vi "PH_VacuumControl.set modified data.vi"(0 "i ref in":refnum<vi>, 2 "i attribute":T1={"GUI Refs"={"Exit"=refnum, "Set Unit"=refnum, "Device found"=refnum, "Busy"=refnum, "State"=refnum, "Delete"=refnum, "Channels"=refnum, "Channel Name"=refnum, "Trend"=refnum, "Logarithmic"=refnum, "Limit reached"=refnum, "Channel Name 1 MT"=refnum, "Channel Name 2 MT"=refnum, "Trend MT"=refnum, "Logarithmic MT"=refnum, "Limit reached MT"=refnum}, "Device found"=FALSE, "Busy"=FALSE, "Selected Unit"=1, "Channels [mbar]"={"Channel 1"=99999.0, "Channel 2"=99999.0, "Channel 3"=99999.0, "Channel 4"=99999.0, "Channel 5"=99999.0, "Channel 6"=99999.0, "Name Channel 1"="", "Name Channel 2"="", "Name Channel 3"="", "Name Channel 4"="", "Name Channel 5"="", "Name Channel 6"="", "Upper Limit"=0.0, "Upper Limit 2"=0.0, "Upper Limit 3"=0.0, "Upper Limit 4"=0.0, "Upper Limit 5"=0.0, "Upper Limit 6"=0.0}, "Channel Names"={"Channel 1"="N/A", "Channel 2"="N/A", "Channel 3"="N/A", "Channel 4"="N/A", "Channel 5"="N/A", "Channel 6"="N/A"}, "Status"=0, "AGCxxx VISA Cluster"={"VISA resource name"="", "VISA Timeout Value (1000 ms)"=1000, "Lock Timeout (1000 ms)"=1000, "MAX Channel (6)"=6}, "Instr Firmware Revision"="N/A", "Service IDs Pressure"={"Channel 1"=-1, "Channel 2"=-1, "Channel 3"=-1, "Channel 4"=-1, "Channel 5"=-1, "Channel 6"=-1}, "Service IDs Limits"={"Channel 1"=-1, "Channel 2"=-1, "Channel 3"=-1, "Channel 4"=-1, "Channel 5"=-1, "Channel 6"=-1}, "Trend"={"Start Point"=timestamp(0 s since 1904-01-01), "Pressures [mbar] Channel 1"=[], "Pressures [mbar] Channel 2"=[], "Pressures [mbar] Channel 3"=[], "Pressures [mbar] Channel 4"=[], "Pressures [mbar] Channel 5"=[], "Pressures [mbar] Channel 6"=[], "Timebase [s]"=[], "Trend Channel"=0, "Start Fit"=0.0, "Trend Channel 1 MT"=0, "Trend Channel 2 MT"=0, "Start or continue Fit MT"=0.0, "Continue or start Fit MT"=0.0, "Datasets strored"=0, "Dataarray Size"=0}, "Running"=FALSE} {"Status" items=["no info", "off/false/out", "on/true/in", "Failure", "Alarm", "Status 1", "Status 2", "Status 3"]; "Channels [mbar]"."Upper Limit 6" format="%.4e"; "Channels [mbar]"."Upper Limit 5" format="%.4e"; "Channels [mbar]"."Upper Limit 4" format="%.4e"; "Channels [mbar]"."Upper Limit 3" format="%.4e"; "Channels [mbar]"."Upper Limit 2" format="%.4e"; "Channels [mbar]"."Upper Limit" format="%.4e"; "Channels [mbar]"."Channel 6" format="%.4e"; "Channels [mbar]"."Channel 5" format="%.4e"; "Channels [mbar]"."Channel 4" format="%.4e"; "Channels [mbar]"."Channel 3" format="%.4e"; "Channels [mbar]"."Channel 2" format="%.4e"; "Channels [mbar]"."Channel 1" format="%.4e"; "Selected Unit" items=["mBar", "Pascal", "Torr"]}, 5 "error in (no error)":errorcluster) -> (14 "i ref out":refnum<vi>, 19 "error out":errorcluster)   [LabVIEW 2014, in "PH_VacuumControl.lvlib"]
doc: "Writes the data into the attribute of an object. Then, the attribute dara are unlocked using the \"release\" method. Prior to calling THIS method, the attribute data must have been locked using the methods \"lock\" or \"get data to modify\".\n\n\nLicense Agreement for this software:\n\nCopyright (C)\nGesellschaft für Schwerionenforschung, GSI\nPlanckstr. 1\n64291 Darmstadt\nGermany\n\nContact: D.Beck@gsi.de \n\nThis program is free software; you can redistribute it and/or modify it under the terms of the GNU General Public License as published by the Free Software Foundation; either version 2 of the license, or (at your option) any later version.\n\nThis program is distributed in the hope that it will be useful, but WITHOUT ANY WARRANTY; without even the implied warranty of MERCHANTABILITY or FITNESS FOR A PARTICULAR PURPOSE. See the GNU General License for more details (http://www.gnu.org).\n\nGesellschaft für Schwerionenforschung, GSI\nPlanckstr. 1, 64291 Darmstadt, Germany\nFor all questions and ideas contact: M.Richter@gsi.de, H.Brand@gsi.de or D.Beck@gsi.de.\nLast update: 17-JUN-2004"
uses:
  PH_VacuumControl.lvlib
  PH_VacuumControl.i attribute.ctl
  PH_VacuumControl.Channels.ctl
  PH_StatusHandler/PH_StatusHandler.Status.ctl
  instr.lib/AGCxxx/AGCxxx/AGCxxx VISA Control.ctl
  CSCore/CSObj/CSObj.lvlib
  instr.lib/AGCxxx/AGCxxx - Driver.lvlib
  PH_StatusHandler/PH_StatusHandler.lvlib
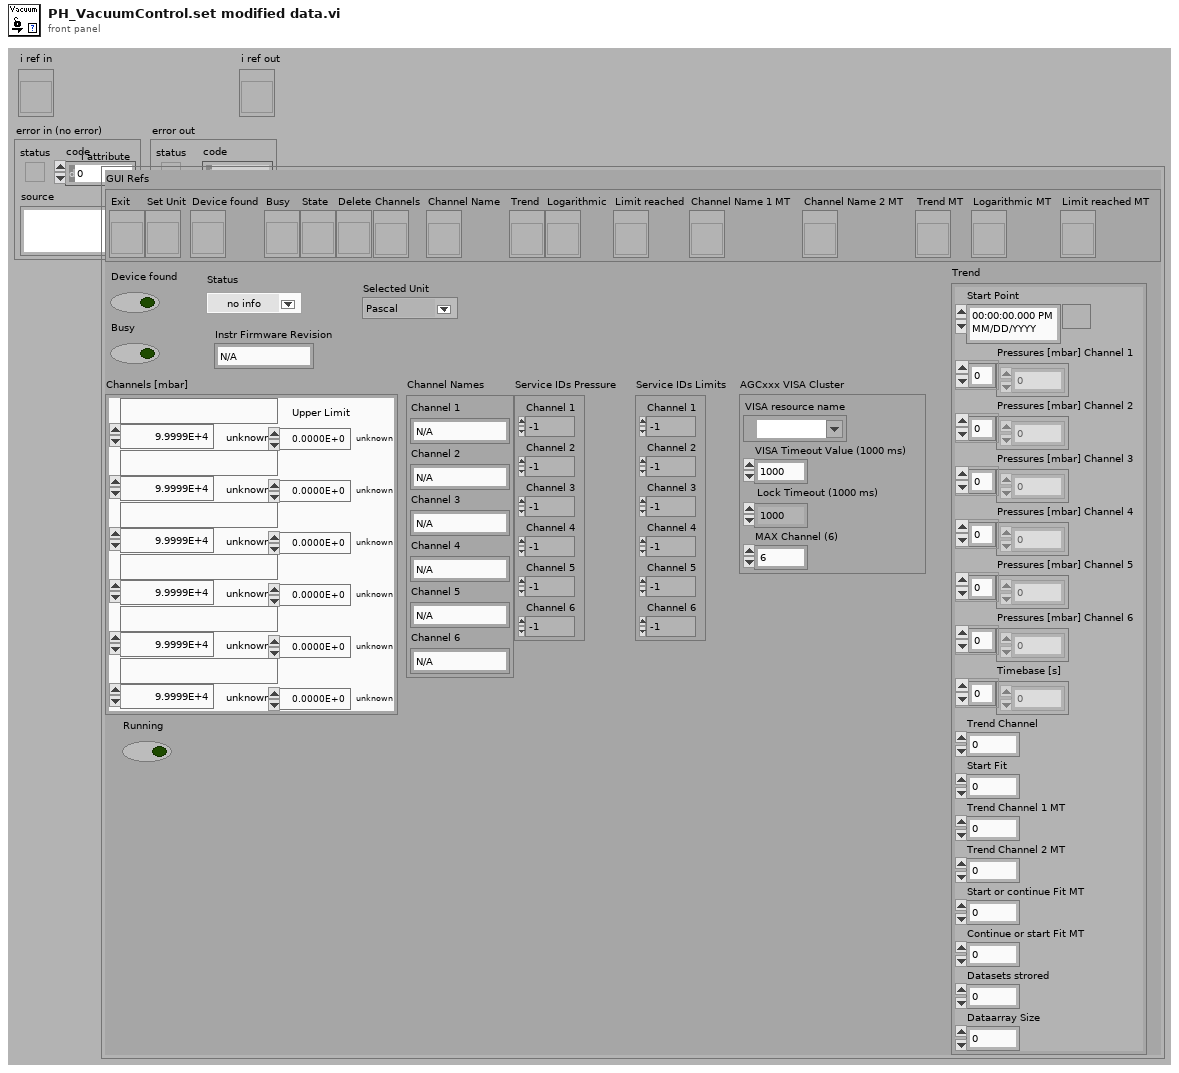
[diagram p1: front panel]
types:
  T1 = typedef "PH_VacuumControl.lvlib/PH_VacuumControl.i attribute.ctl" = cluster{"GUI Refs":cluster{"Exit":refnum<vi>, "Set Unit":refnum<vi>, "Device found":refnum<vi>, "Busy":refnum<vi>, "State":refnum<vi>, "Delete":refnum<vi>, "Channels":refnum<vi>, "Channel Name":refnum<vi>, "Trend":refnum<vi>, "Logarithmic":refnum<vi>, "Limit reached":refnum<vi>, "Channel Name 1 MT":refnum<vi>, "Channel Name 2 MT":refnum<vi>, "Trend MT":refnum<vi>, "Logarithmic MT":refnum<vi>, "Limit reached MT":refnum<vi>}, "Device found":bool, "Busy":bool, "Selected Unit":i32, "Channels [mbar]":T2, "Channel Names":cluster{"Channel 1":string, "Channel 2":string, "Channel 3":string, "Channel 4":string, "Channel 5":string, "Channel 6":string}, "Status":T3, "AGCxxx VISA Cluster":T4, "Instr Firmware Revision":string, "Service IDs Pressure":cluster{"Channel 1":i32, "Channel 2":i32, "Channel 3":i32, "Channel 4":i32, "Channel 5":i32, "Channel 6":i32}, "Service IDs Limits":cluster{"Channel 1":i32, "Channel 2":i32, "Channel 3":i32, "Channel 4":i32, "Channel 5":i32, "Channel 6":i32}, "Trend":cluster{"Start Point":timestamp, "Pressures [mbar] Channel 1":dbl[], "Pressures [mbar] Channel 2":dbl[], "Pressures [mbar] Channel 3":dbl[], "Pressures [mbar] Channel 4":dbl[], "Pressures [mbar] Channel 5":dbl[], "Pressures [mbar] Channel 6":dbl[], "Timebase [s]":i32[], "Trend Channel":u16, "Start Fit":dbl, "Trend Channel 1 MT":u16, "Trend Channel 2 MT":u16, "Start or continue Fit MT":dbl, "Continue or start Fit MT":dbl, "Datasets strored":i32, "Dataarray Size":i32}, "Running":bool}
  T2 = typedef "PH_VacuumControl.lvlib/PH_VacuumControl.Channels.ctl" = cluster{"Channel 1":dbl, "Channel 2":dbl, "Channel 3":dbl, "Channel 4":dbl, "Channel 5":dbl, "Channel 6":dbl, "Name Channel 1":string, "Name Channel 2":string, "Name Channel 3":string, "Name Channel 4":string, "Name Channel 5":string, "Name Channel 6":string, "Upper Limit":dbl, "Upper Limit 2":dbl, "Upper Limit 3":dbl, "Upper Limit 4":dbl, "Upper Limit 5":dbl, "Upper Limit 6":dbl}
  T3 = typedef "PH_StatusHandler.lvlib/PH_StatusHandler.Status.ctl" = i16
  T4 = typedef "AGCxxx - Driver.lvlib/AGCxxx VISA Control.ctl" = cluster{"VISA resource name":refnum<visa-resource-name>, "VISA Timeout Value (1000 ms)":u32, "Lock Timeout (1000 ms)":u32, "MAX Channel (6)":i32}
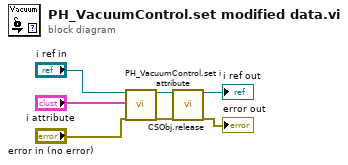
[diagram p0: block diagram]
diagram:
  n1 = call "PH_VacuumControl.set i attribute.vi"("i ref in"="i ref in", "i attribute"="i attribute", "error in (no error)"="error in (no error)") -> ("i ref out"=w4:refnum<vi>, "error out"=w3:errorcluster)  [unwired: 15 in]
  n2 = call "CSObj.release.vi"("i ref in"=w4, "error in (no error)"=w3) -> ("i ref out"=→"i ref out":refnum<vi>, "error out"=→"error out":errorcluster)  [unwired: 16 in]
